vi "Template.vi"() -> ()   [LabVIEW 2013]
uses:
  Public_Ctl/Motor_Parameters.ctl
  <vilib>/Motion/PropertyNodes/nimc.createStraightLineMoveInstance.axis.vi
  <vilib>/Motion/PropertyNodes/nimc.destroyInterfaceInstance.vi
  <resource>/objmgr/nimotion.rc
panel:
  in  "table":refnum<k21>
  in  "coordinate":refnum<k21>
  in  "Motion Parameters":T1={"position"=1000.0, "velocity"=1000.0, "acceleration"=10000.0, "deceleration"=10000.0, "accel. jerk"=10000.0, "decel. jerk"=10000.0}
  in  "axis":refnum<k21>
  out "error out":errorcluster
  in  "error in (no error)":errorcluster
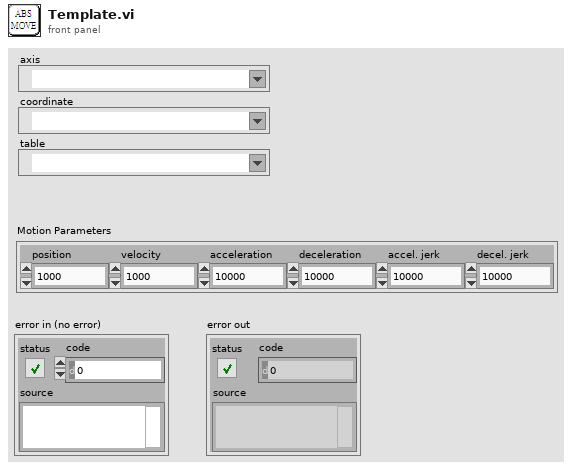
[diagram p1: front panel]
types:
  T1 = typedef "Motor_Parameters.ctl" = cluster{"position":dbl, "velocity":dbl, "acceleration":dbl, "deceleration":dbl, "accel. jerk":dbl, "decel. jerk":dbl}
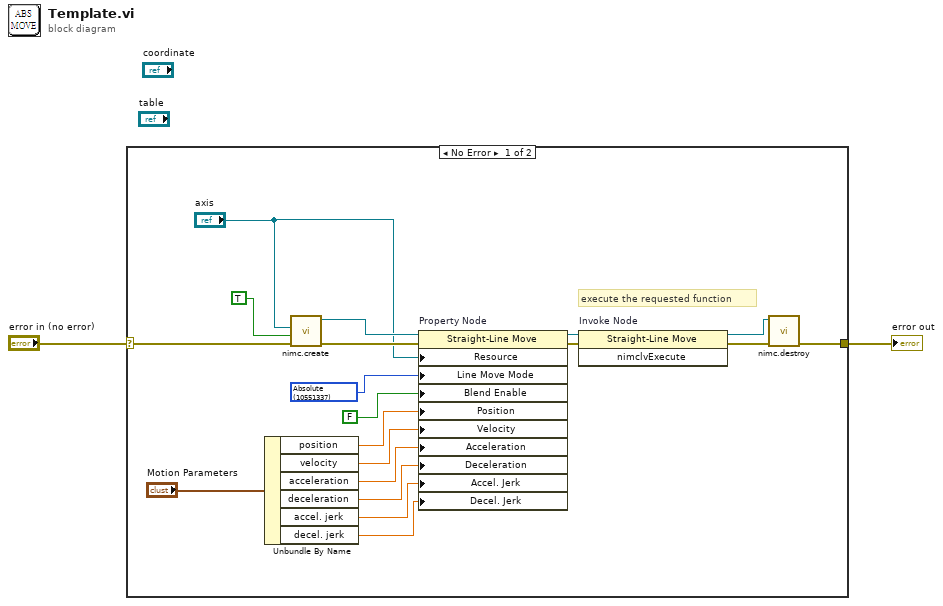
[diagram p0: block diagram]
diagram:
  n1 = case shown="No Error" "error in (no error)" {
    selector: "error in (no error)" -> [w3 w22]
    tunnel: [w15 w22] -> w2
    frame No Error {
      w5 = 10551337 items=["Relative"=10551344, "Absolute"=10551337, "Relative To Capture"=10551345, "Velocity"=10551346, "Polyline"=11600101] ("line move mode")
      # "execute the requested function"
      n2 = Unbundle By Name("Motion Parameters") -> ("position"=w11:dbl, "velocity"=w10:dbl, "acceleration"=w9:dbl, "deceleration"=w8:dbl, "accel. jerk"=w7:dbl, "decel. jerk"=w6:dbl)
      n3 = call-poly <vilib>:"nimc.create.vi"("error in"=w3, "async?"=TRUE ("execute asynchronously?"), "axis"="axis") -> ("error out"=w18:errorcluster, "line"=w13:refnum<k20>)  [unwired: 6 in, 1 out]
      n4 = property on="Property Node" class="Straight-Line Move"(reference=w13, error in=w18, "Resource"="axis", "Line Move Mode"=w5, "Blend Enable"=FALSE ("blend enable"), "Position"=w11, "Velocity"=w10, "Acceleration"=w9, "Deceleration"=w8, "Accel. Jerk"=w7, "Decel. Jerk"=w6) -> (reference out=w21:refnum<k20>, error out=w20:errorcluster)
      n5 = invoke on="Invoke Node" class="Straight-Line Move" method="nimclvExecute"(reference=w21, error in=w20) -> (reference out=w17:refnum<k20>, error out=w16:errorcluster)  [unwired: 1 in, 1 out]
      n6 = call-poly <vilib>:"nimc.destroy.vi"("error in"=w16, "motion handle"=w17) -> ("error out"=w15:errorcluster)  [unwired: 9 in]
    }
    frame Error {
    }
  }
  "error out" <- w2
